vi "Create.vi"(8 "error in (no error)":errorcluster, 11 "Map in":refnum<class "Map.lvclass">) -> (0 "error out":errorcluster, 3 "Map out":refnum<class "Map.lvclass">)   [LabVIEW 2019, in "Map.lvclass"]
uses:
  Map.lvclass
  TCP Packet/Packet.lvclass
  TCP Packet/packet type STYP.ctl
  C:/projects/labview_multiplayer_snake/Main Codeline/Software/Code/Shared/TCP/JSONPayload/JSONPayload.lvclass
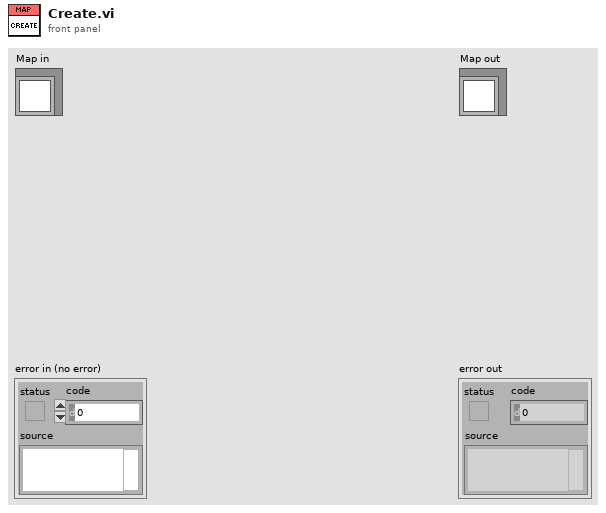
[diagram p1: front panel]
types:
  T1 = typedef "Packet.lvclass/packet type STYP.ctl" = enum16{"Connect", "Disconnect", "Direction", "Score", "Map"}
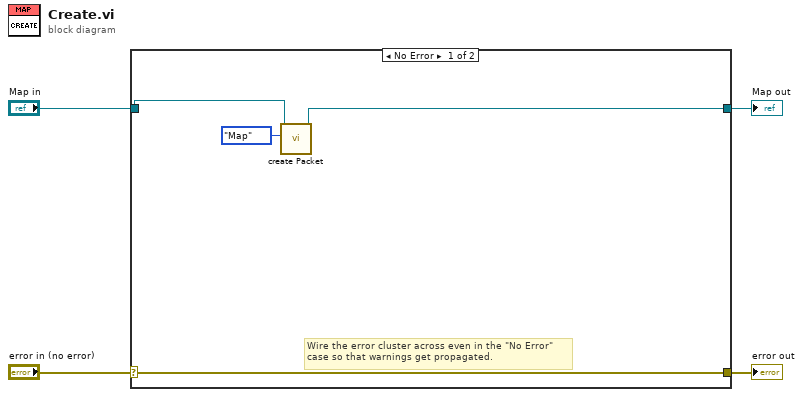
[diagram p0: block diagram]
diagram:
  n1 = case shown="No Error" "error in (no error)" {
    selector: "error in (no error)" -> [w8 w10]
    tunnel: [w8 w10] -> w3
    tunnel: [w6 w9] -> w1
    tunnel: "Map in" -> [w7 w9]
    frame No Error {
      # "Wire the error cluster across even in the \"No Error\"\ncase so that warnings get propagated."
      n2 = call "create Packet.vi"("Packet Type"=packet_type_STYP."Map", "Packet in"=w7) -> ("Packet out"=w6:refnum<class "Packet.lvclass">)  [unwired: 8 in, 1 out]
    }
    frame Error {
    }
  }
  "error out" <- w3
  "Map out" <- w1
